vi "ComputeSampleData.vi"(9 "MeasuredFlow":dbl, 10 "MeasuredDeltaPressure":dbl, 11 "UserFilledData":T2) -> (3 "MeasureData":T1)   [LabVIEW 2012]
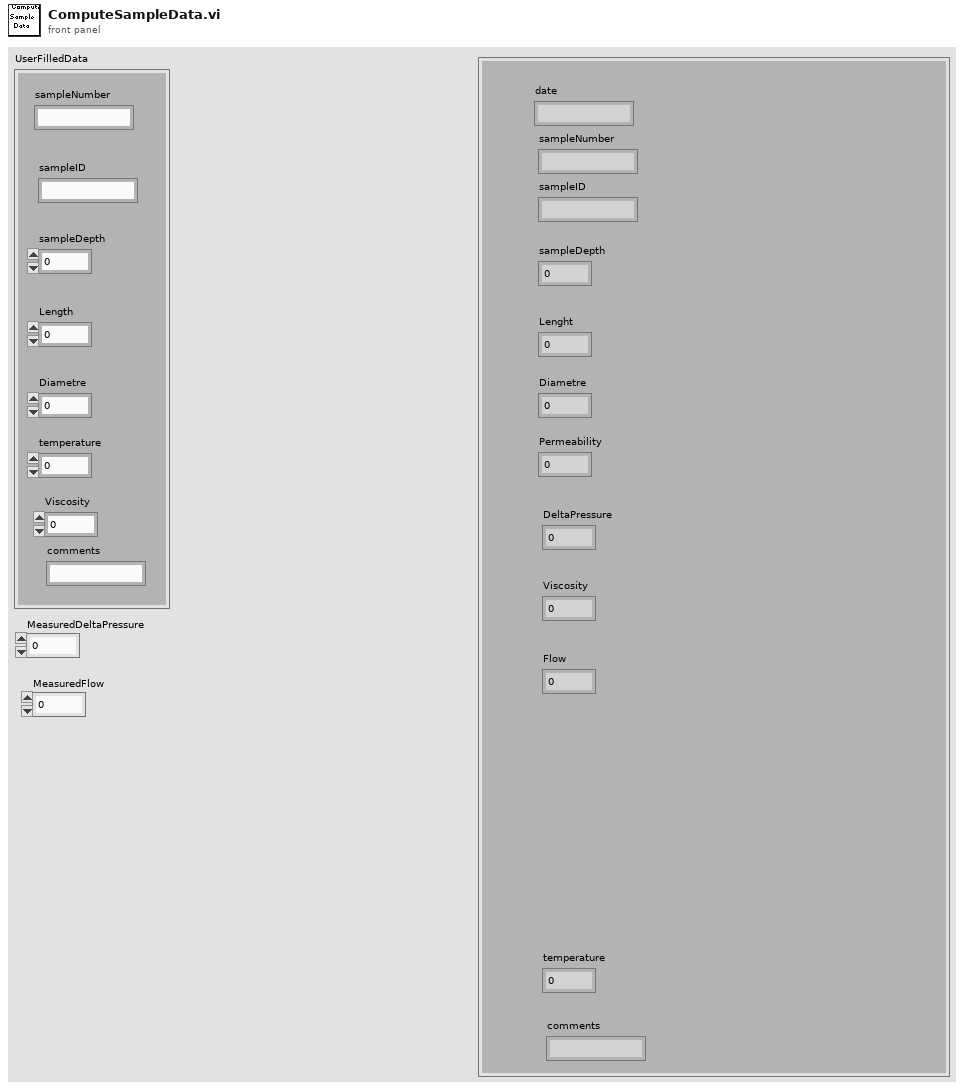
[diagram p1: front panel]
types:
  T1 = cluster{"date":string, "sampleNumber":string, "sampleID":string, "sampleDepth":dbl, "Lenght":dbl, "Permeability":dbl, "Diametre":dbl, "DeltaPressure":dbl, "Viscosity":dbl, "Flow":dbl, "temperature":dbl, "comments":string}
  T2 = cluster{"sampleNumber":string, "sampleID":string, "sampleDepth":dbl, "Length":dbl, "Diametre":dbl, "temperature":dbl, "comments":string, "Viscosity":dbl}
  T3 = cluster{string, "sampleNumber":string, "sampleID":string, "sampleDepth":dbl, "Length":dbl, "Diametre":dbl, dbl, "MeasuredDeltaPressure":dbl, "Viscosity":dbl, "MeasuredFlow":dbl, "temperature":dbl, "comments":string}
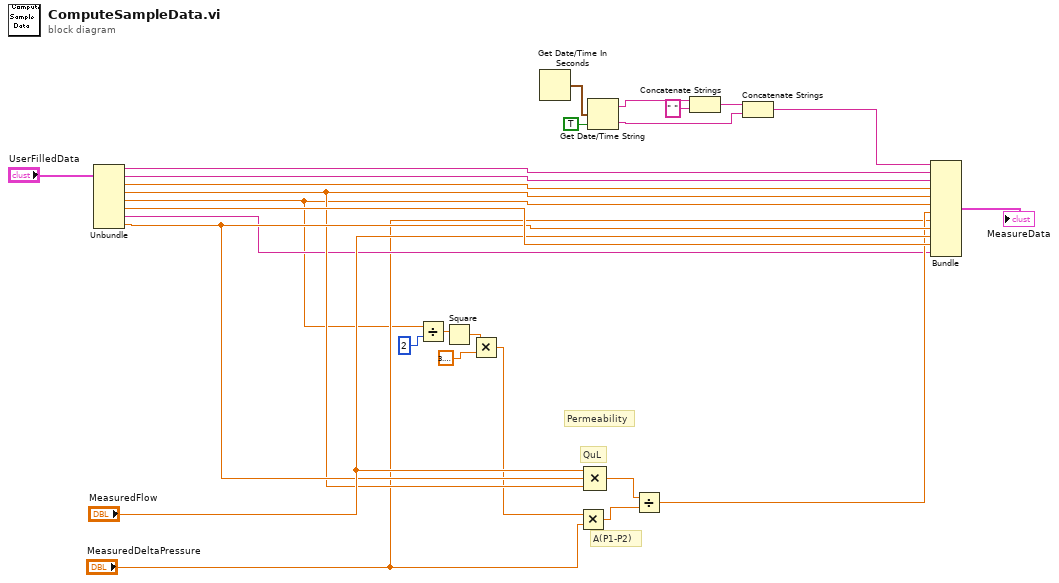
[diagram p0: block diagram]
diagram:
  # "A(P1-P2)"
  # "QuL"
  # "Permeability"
  n1 = Unbundle("UserFilledData") -> ("sampleNumber"=w26:string, "sampleID"=w25:string, "sampleDepth"=w24:dbl, "Length"=w12:dbl, "Diametre"=w5:dbl, "temperature"=w15:dbl, "comments"=w8:string, "Viscosity"=w13:dbl)
  n2 = Divide(x=w5, y=2) -> (x/y=w4:dbl)
  n3 = Square(x=w4) -> (x^2=w2:dbl)
  n4 = Multiply(x=w2, y=3.141592653589793) -> (x*y=w1:dbl)
  n5 = Get Date/Time In Seconds() -> (seconds since 1Jan1904=w22:timestamp)
  n6 = Multiply(x=w1, y="MeasuredDeltaPressure") -> (x*y=w10:dbl)
  n7 = Compound Arithmetic op=MULTIPLY("MeasuredFlow", w13, w12) -> (w11:dbl)
  n8 = Get Date/Time String(seconds (now)=w22, want seconds? (F)=TRUE) -> (date string=w21:string, time string=w18:string)  [unwired: 1 in]
  n9 = Divide(x=w11, y=w10) -> (x/y=w9:dbl)
  n10 = Concatenate Strings(w21, " " ("string")) -> (w19:string)
  n11 = Concatenate Strings(w19, w18) -> (w17:string)
  n12 = Bundle(w17, "sampleNumber"=w26, "sampleID"=w25, "sampleDepth"=w24, "Length"=w12, "Diametre"=w5, w9, "MeasuredDeltaPressure"="MeasuredDeltaPressure", "Viscosity"=w13, "MeasuredFlow"="MeasuredFlow", "temperature"=w15, "comments"=w8) -> (→"MeasureData":T3)  [unwired: 1 in]
